vi "var global.vi"(6 "Action":enum16{"Set", "Get"}(ring), 11 "input":T2={"Play"=FALSE, "Format (44kHz, 16Bit, stereo)"={"Rate"=48000, "Bits"=16, "Channels"=2}, "Buffer Config"={"# buffers"=4, "Buffer size"=600, "unit (ms)"=enum."Samples"}, "idev"=0, "millisec to wait"=1000}) -> (3 "output":T1={"Play"=FALSE, "Format (44kHz, 16Bit, stereo)"={"Rate"=48000, "Bits"=16, "Channels"=2}, "Buffer Config"={"# buffers"=4, "Buffer size"=600, "unit (ms)"=enum."Samples"}, "idev"=0, "millisec to wait"=1000})   [LabVIEW 2018]
uses:
  Control 3.ctl
  Control 4.ctl
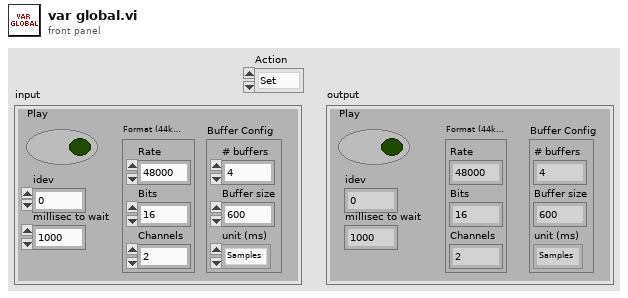
[diagram p1: front panel]
types:
  T1 = typedef "Control 4.ctl" = cluster{"Play":bool, "Format (44kHz, 16Bit, stereo)":cluster{"Rate":i32, "Bits":i32, "Channels":u32}, "Buffer Config":cluster{"# buffers":i32, "Buffer size":i32, "unit (ms)":enum16{"time (ms)", "Samples"}}, "idev":u32, "millisec to wait":u32}
  T2 = typedef "Control 3.ctl" = cluster{"Play":bool, "Format (44kHz, 16Bit, stereo)":cluster{"Rate":i32, "Bits":i32, "Channels":u32}, "Buffer Config":cluster{"# buffers":i32, "Buffer size":i32, "unit (ms)":enum16{"time (ms)", "Samples"}}, "idev":u32, "millisec to wait":u32}
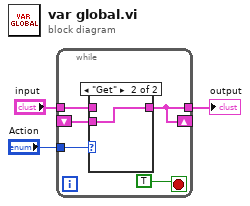
[diagram p0: block diagram]
diagram:
  n1 = while {
    tunnel: "Action" -> [w8]
    tunnel: "input" -> [w7]
    shift-right: [w6] -> _
    shift-left: _ -> [w5]
    tunnel: [w6] -> w1
    stop <- TRUE stop-if-true
    n2 = case shown="\"Get\"" w8 {
      tunnel: w7 -> [w9 _]
      tunnel: [w9 w10] -> w6
      tunnel: w5 -> [_ w10]
      frame "Set", Default {
      }
      frame "Get" {
      }
    }
  }
  "output" <- w1
